vi "HigakiBSetU-I_Wrapper.vi"(0 "File Array":string[](array[string])=["C:\\CuspControl\\GPIB and Network\\Positron\\HigakiB.txt", "6723"], 1 "Input Values":dbl[](array[numeric])=[0.0]) -> ()   [LabVIEW 2018]
panel:
  out "x-y":u32=59
  out "Device name":string[](array[string])=["GPIB0::8::INSTR"]
  out "Set Values":dbl[](array[numeric])=[200.0, 60.0, 60.0, 0.0]
  out "Enable\nHigaki B?":bool
  out "error out":errorcluster
  out "Current String":string="#2 ISET 60.000000\r\n"
  out "Voltage string":string="#2 VSET 0.000000\r\n"
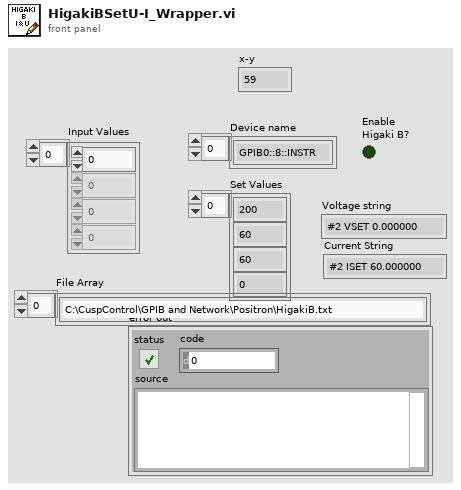
[diagram p1: front panel]
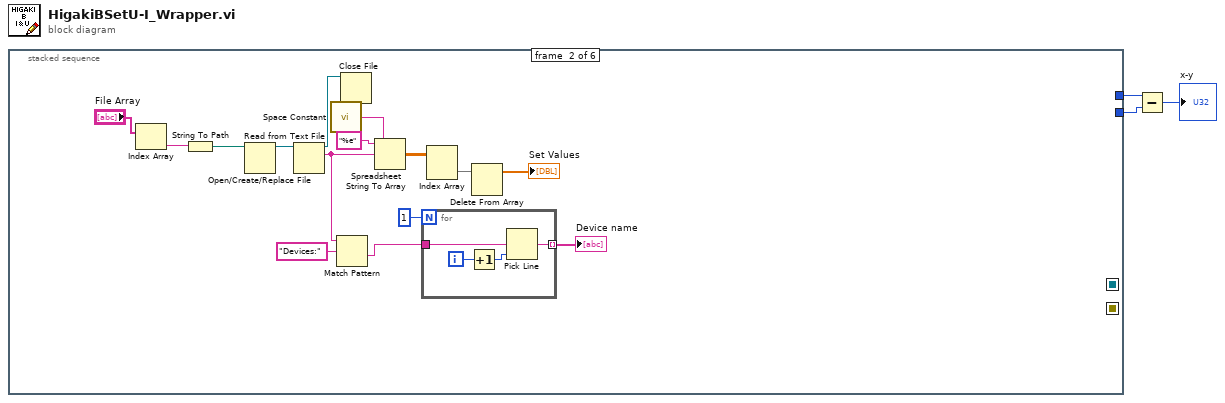
[diagram p0: block diagram]
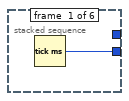
[diagram p2: hidden frame]
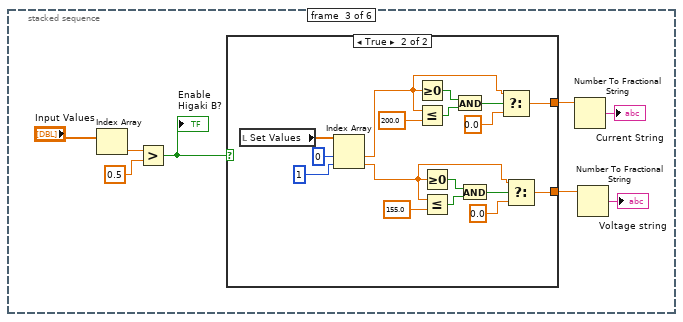
[diagram p3: hidden frame]
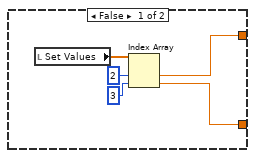
[diagram p4: hidden frame]
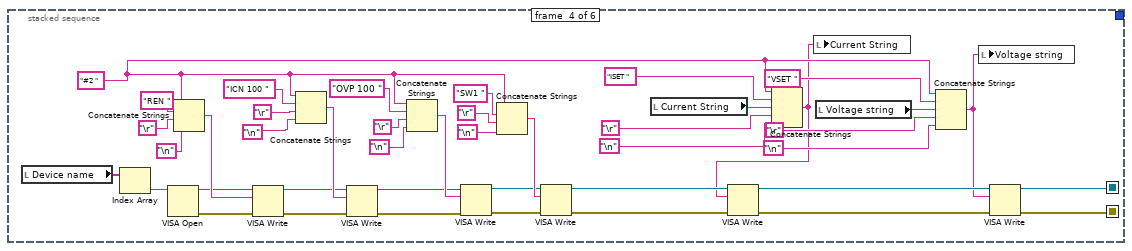
[diagram p5: hidden frame]
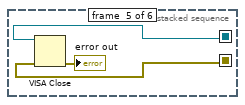
[diagram p6: hidden frame]
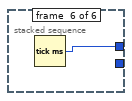
[diagram p7: hidden frame]
diagram:
  n1 = stacked-sequence {
    seq-local: [_ _ _ w58 _ _] -> [_ _ _ _ w99 _]
    seq-local: [_ _ _ w57 _ _] -> [_ _ _ _ w98 _]
    tunnel: [w4 _ _ _ _ _] -> w2
    tunnel: [_ _ _ _ _ w100] -> w3
    frame #0 {
      n2 = Tick Count (ms)() -> (millisecond timer value=w4:u32)
    }
    frame #1 {
      n3 = Index Array(array="File Array") -> (element=w10:string)  [unwired: 1 in]
      n4 = String To Path(string=w10) -> (path=w8:path)
      n5 = Open/Create/Replace File(file path (use dialog)=w8) -> (refnum out=w7:refnum<file>)  [unwired: 5 in, 2 out]
      n6 = Read from Text File(file (use dialog)=w7) -> (refnum out=w5:refnum<file>, text=w16:string)  [unwired: 3 in, 2 out]
      n7 = call <vilib>:"Space Constant.vi"() -> ("String"=w18:string)
      n8 = Match Pattern(string=w16, regular expression="Devices:") -> (after substring=w14:string)  [unwired: 1 in, 3 out]
      n9 = Close File(refnum=w5) -> ()  [unwired: 1 in, 2 out]
      n10 = Spreadsheet String To Array(delimiter (Tab)=w18, format string="%e", spreadsheet string=w16) -> (array=w17:dbl[][])  [unwired: 1 in]
      n11 = for {
        N: 1 -> [_]
        tunnel: w14 -> [w21]
        tunnel: [w20] -> w12 mode=indexing
        i -> [w23]
        n12 = Increment(x=w23) -> (x+1=w22:i32)
        n13 = Pick Line(multi-line string=w21, line index=w22) -> (output string=w20:string)  [unwired: 1 in]
      }
      "Device name" <- w12
      n14 = Index Array(array=w17) -> (element=w11:dbl[])  [unwired: 2 in]
      n15 = Delete From Array(array=w11) -> (array with subset deleted=→"Set Values":dbl[])  [unwired: 2 in, 1 out]
    }
    frame #2 {
      n16 = Index Array(array="Input Values") -> (element=w25:dbl)  [unwired: 1 in]
      n17 = Greater?(x=w25, y=0.5) -> (0:w30:bool)
      "Enable\nHigaki B?" <- w30
      n18 = case shown="True" w30 {
        tunnel: [w33 w43] -> w28
        tunnel: [w32 w42] -> w26
        frame False {
          n19 = local read "Set Values"() -> (w36:dbl[])
          n20 = Index Array(array=w36, index #1=2 ("index"), index #2=3 ("index")) -> (element #1=w33:dbl, element #2=w32:dbl)
        }
        frame True {
          n21 = local read "Set Values"() -> (w41:dbl[])
          n22 = Index Array(array=w41, index #1=0 ("index"), index #2=1 ("index")) -> (element #1=w38:dbl, element #2=w37:dbl)
          n23 = Greater Or Equal To 0?(x=w38) -> (x >= 0?=w44:bool)
          n24 = Less Or Equal?(x=w38, y=200.0) -> (x <= y?=w45:bool)
          n25 = Greater Or Equal To 0?(x=w37) -> (x >= 0?=w53:bool)
          n26 = Less Or Equal?(x=w37, y=155.0) -> (x <= y?=w52:bool)
          n27 = And(x=w44, y=w45) -> (x .and. y?=w47:bool)
          n28 = And(x=w53, y=w52) -> (x .and. y?=w50:bool)
          n29 = Select(t=w38, s=w47, f=0.0) -> (s? t:f=w43:dbl)
          n30 = Select(t=w37, s=w50, f=0.0) -> (s? t:f=w42:dbl)
        }
      }
      n31 = Number To Fractional String(number=w28) -> (F-format string=→"Current String":string)  [unwired: 3 in]
      n32 = Number To Fractional String(number=w26) -> (F-format string=→"Voltage string":string)  [unwired: 3 in]
    }
    frame #3 {
      w74 = "#2 "
      n33 = local read "Device name"() -> (w55:string[])
      n34 = Index Array(array=w55) -> (element=w54:string)  [unwired: 1 in]
      n35 = VISA Open(VISA resource name=w54) -> (VISA resource name=w62:refnum<visa-resource-name>, error out=w63:errorcluster)  [unwired: 4 in]
      n36 = Concatenate Strings(w74, "REN " ("write buffer"), "\r", "\n") -> (w75:string)
      n37 = VISA Write(VISA resource name=w62, write buffer=w75, error in (no error)=w63) -> (VISA resource name out=w73:refnum<visa-resource-name>, error out=w68:errorcluster)  [unwired: 1 out]
      n38 = Concatenate Strings(w74, "ICN 100 " ("write buffer"), "\r", "\n") -> (w80:string)
      n39 = VISA Write(VISA resource name=w73, write buffer=w80, error in (no error)=w68) -> (VISA resource name out=w72:refnum<visa-resource-name>, error out=w67:errorcluster)  [unwired: 1 out]
      n40 = Concatenate Strings(w74, "OVP 100 " ("write buffer"), "\r", "\n") -> (w83:string)
      n41 = VISA Write(VISA resource name=w72, write buffer=w83, error in (no error)=w67) -> (VISA resource name out=w71:refnum<visa-resource-name>, error out=w66:errorcluster)  [unwired: 1 out]
      n42 = Concatenate Strings(w74, "SW1 " ("write buffer"), "\r", "\n") -> (w86:string)
      n43 = VISA Write(VISA resource name=w71, write buffer=w86, error in (no error)=w66) -> (VISA resource name out=w70:refnum<visa-resource-name>, error out=w65:errorcluster)  [unwired: 1 out]
      n44 = local read "Current String"() -> (w61:string)
      n45 = Concatenate Strings(w74, "ISET " ("write buffer"), w61, "\r", "\n") -> (w60:string)
      n46 = VISA Write(VISA resource name=w70, write buffer=w60, error in (no error)=w65) -> (VISA resource name out=w69:refnum<visa-resource-name>, error out=w64:errorcluster)  [unwired: 1 out]
      n47 = local write "Current String"(w60) -> ()
      n48 = local read "Voltage string"() -> (w59:string)
      n49 = Concatenate Strings(w74, "VSET " ("write buffer"), w59, "\r", "\n") -> (w56:string)
      n50 = local write "Voltage string"(w56) -> ()
      n51 = VISA Write(VISA resource name=w69, write buffer=w56, error in (no error)=w64) -> (VISA resource name out=w58:refnum<visa-resource-name>, error out=w57:errorcluster)  [unwired: 1 out]
    }
    frame #4 {
      n52 = VISA Close(VISA resource name=w99, error in (no error)=w98) -> (error out=→"error out":errorcluster)
    }
    frame #5 {
      n53 = Tick Count (ms)() -> (millisecond timer value=w100:u32)
    }
  }
  n54 = Subtract(x=w3, y=w2) -> (x-y=→"x-y":u32)
